vi "DumpToDashboard.vi"   [LabVIEW 2012]
uses:
  <vilib>/Rock Robotics/WPI/Joystick/WPI_JoystickGetSetRefNum.vi
types:
  T1 = typedef "WPI_JoystickDevRef.ctl" = cluster{"Device":T2}
  T2 = typedef "WPI_JoystickDeviceEnum.ctl" = enum16{"USB 1", "USB 2", "USB 3", "USB 4", "Kinect 1", "Kinect 2"}
  T3 = typedef "WPI_JoystickButtonState.ctl" = cluster{"Button 1":bool, "Button 2":bool, "Button 3":bool, "Button 4":bool, "Button 5":bool, "Button 6":bool, "Button 7":bool, "Button 8":bool, "Button 9":bool, "Button 10":bool, "Button 11":bool, "Button 12":bool}
  T4 = cluster{"axis 1 (x)":dbl, "axis 2 (y)":dbl, "axis 3 (throttle)":dbl, "axis 4":dbl, "axis 5":dbl, "axis 6":dbl}
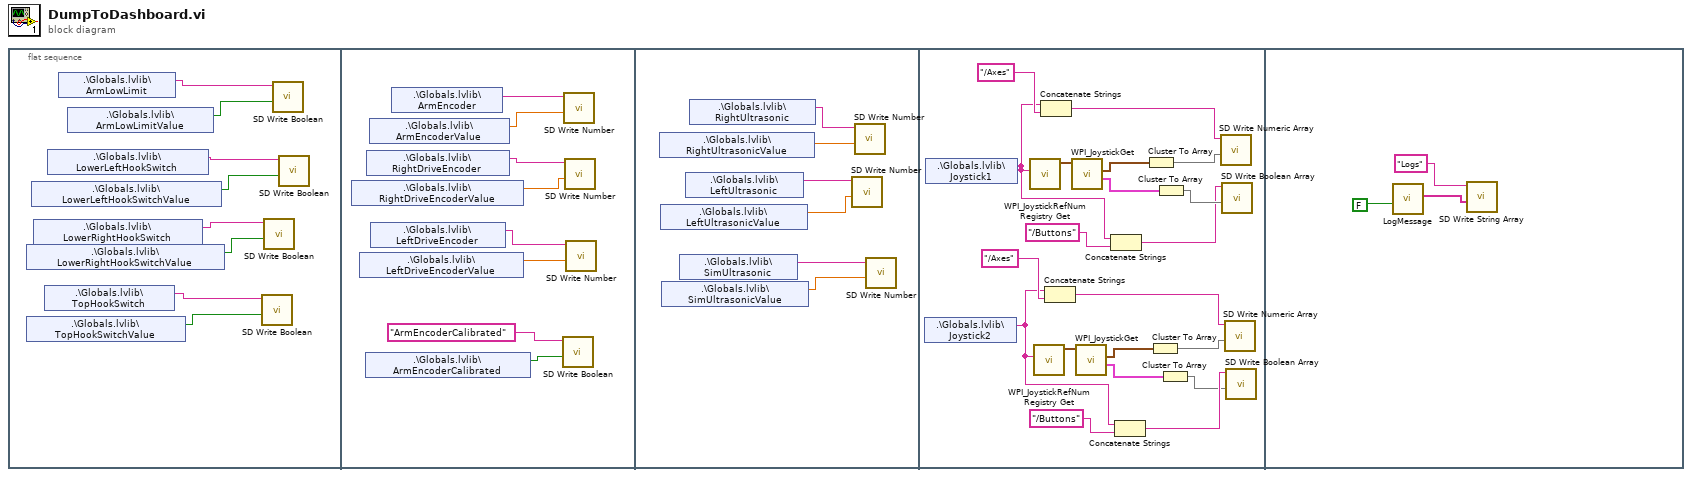
[diagram p0: block diagram]
diagram:
  n1 = flat-sequence {
    frame #0 {
      n2 = shared-variable ".\\Globals.lvlib\\LowerRightHookSwitchValue"() -> (w2:bool)  [unwired: 1 in, 1 out]
      n3 = shared-variable ".\\Globals.lvlib\\TopHookSwitchValue"() -> (w1:bool)  [unwired: 1 in, 1 out]
      n4 = shared-variable ".\\Globals.lvlib\\LowerLeftHookSwitchValue"() -> (w3:bool)  [unwired: 1 in, 1 out]
      n5 = shared-variable ".\\Globals.lvlib\\LowerRightHookSwitch"() -> (w6:string)  [unwired: 1 in, 1 out]
      n6 = shared-variable ".\\Globals.lvlib\\TopHookSwitch"() -> (w7:string)  [unwired: 1 in, 1 out]
      n7 = shared-variable ".\\Globals.lvlib\\LowerLeftHookSwitch"() -> (w5:string)  [unwired: 1 in, 1 out]
      n8 = shared-variable ".\\Globals.lvlib\\ArmLowLimit"() -> (w8:string)  [unwired: 1 in, 1 out]
      n9 = shared-variable ".\\Globals.lvlib\\ArmLowLimitValue"() -> (w4:bool)  [unwired: 1 in, 1 out]
      n10 = call <vilib>:"SD Write Boolean.vi"("Boolean"=w1, "Name"=w7) -> ()  [unwired: 8 in, 2 out]
      n11 = call <vilib>:"SD Write Boolean.vi"("Boolean"=w2, "Name"=w6) -> ()  [unwired: 8 in, 2 out]
      n12 = call <vilib>:"SD Write Boolean.vi"("Boolean"=w4, "Name"=w8) -> ()  [unwired: 8 in, 2 out]
      n13 = call <vilib>:"SD Write Boolean.vi"("Boolean"=w3, "Name"=w5) -> ()  [unwired: 8 in, 2 out]
    }
    frame #1 {
      n14 = shared-variable ".\\Globals.lvlib\\RightDriveEncoderValue"() -> (w13:dbl)  [unwired: 1 in, 1 out]
      n15 = shared-variable ".\\Globals.lvlib\\LeftDriveEncoderValue"() -> (w11:dbl)  [unwired: 1 in, 1 out]
      n16 = shared-variable ".\\Globals.lvlib\\ArmEncoderCalibrated"() -> (w10:bool)  [unwired: 1 in, 1 out]
      n17 = shared-variable ".\\Globals.lvlib\\RightDriveEncoder"() -> (w14:string)  [unwired: 1 in, 1 out]
      n18 = shared-variable ".\\Globals.lvlib\\ArmEncoderValue"() -> (w16:dbl)  [unwired: 1 in, 1 out]
      n19 = shared-variable ".\\Globals.lvlib\\LeftDriveEncoder"() -> (w12:string)  [unwired: 1 in, 1 out]
      n20 = shared-variable ".\\Globals.lvlib\\ArmEncoder"() -> (w15:string)  [unwired: 1 in, 1 out]
      n21 = call <vilib>:"SD Write Boolean.vi"("Boolean"=w10, "Name"="ArmEncoderCalibrated") -> ()  [unwired: 8 in, 2 out]
      n22 = call <vilib>:"SD Write Number.vi"("Numeric"=w16, "Name"=w15) -> ()  [unwired: 8 in, 2 out]
      n23 = call <vilib>:"SD Write Number.vi"("Numeric"=w13, "Name"=w14) -> ()  [unwired: 8 in, 2 out]
      n24 = call <vilib>:"SD Write Number.vi"("Numeric"=w11, "Name"=w12) -> ()  [unwired: 8 in, 2 out]
    }
    frame #2 {
      n25 = shared-variable ".\\Globals.lvlib\\RightUltrasonicValue"() -> (w21:dbl)  [unwired: 1 in, 1 out]
      n26 = shared-variable ".\\Globals.lvlib\\LeftUltrasonicValue"() -> (w19:dbl)  [unwired: 1 in, 1 out]
      n27 = shared-variable ".\\Globals.lvlib\\SimUltrasonicValue"() -> (w17:dbl)  [unwired: 1 in, 1 out]
      n28 = shared-variable ".\\Globals.lvlib\\SimUltrasonic"() -> (w18:string)  [unwired: 1 in, 1 out]
      n29 = shared-variable ".\\Globals.lvlib\\LeftUltrasonic"() -> (w20:string)  [unwired: 1 in, 1 out]
      n30 = shared-variable ".\\Globals.lvlib\\RightUltrasonic"() -> (w22:string)  [unwired: 1 in, 1 out]
      n31 = call <vilib>:"SD Write Number.vi"("Numeric"=w19, "Name"=w20) -> ()  [unwired: 8 in, 2 out]
      n32 = call <vilib>:"SD Write Number.vi"("Numeric"=w21, "Name"=w22) -> ()  [unwired: 8 in, 2 out]
      n33 = call <vilib>:"SD Write Number.vi"("Numeric"=w17, "Name"=w18) -> ()  [unwired: 8 in, 2 out]
    }
    frame #3 {
      n34 = shared-variable ".\\Globals.lvlib\\Joystick2"() -> (w23:string)  [unwired: 1 in, 1 out]
      n35 = shared-variable ".\\Globals.lvlib\\Joystick1"() -> (w33:string)  [unwired: 1 in, 1 out]
      n36 = call <vilib>:"WPI_JoystickRefNum Registry Get.vi"("refnum name"=w33) -> ("JoystickDevRef"=w42:T1)  [unwired: 1 in, 9 out]
      n37 = call <vilib>:"WPI_JoystickRefNum Registry Get.vi"("refnum name"=w23) -> ("JoystickDevRef"=w24:T1)  [unwired: 1 in, 9 out]
      n38 = Concatenate Strings(w33, "/Axes") -> (w37:string)
      n39 = Concatenate Strings(w23, "/Axes") -> (w29:string)
      n40 = call <vilib>:"WPI_JoystickGet.vi"("JoystickDevRef"=w42) -> ("Buttons"=w40:T3, "Axes"=w41:T4)  [unwired: 1 in, 4 out]
      n41 = call <vilib>:"WPI_JoystickGet.vi"("JoystickDevRef"=w24) -> ("Buttons"=w26:T3, "Axes"=w25:T4)  [unwired: 1 in, 4 out]
      n42 = Concatenate Strings(w33, "/Buttons") -> (w34:string)
      n43 = Concatenate Strings(w23, "/Buttons") -> (w32:string)
      n44 = Cluster To Array(cluster=w41) -> (array=w39:dbl[])
      n45 = Cluster To Array(cluster=w25) -> (array=w27:dbl[])
      n46 = Cluster To Array(cluster=w40) -> (array=w36:bool[])
      n47 = Cluster To Array(cluster=w26) -> (array=w30:bool[])
      n48 = call <vilib>:"SD Write Numeric Array.vi"("Numeric Array"=w39, "Name"=w37) -> ()  [unwired: 8 in, 2 out]
      n49 = call <vilib>:"SD Write Boolean Array.vi"("Boolean Array"=w36, "Name"=w34) -> ()  [unwired: 8 in, 2 out]
      n50 = call <vilib>:"SD Write Numeric Array.vi"("Numeric Array"=w27, "Name"=w29) -> ()  [unwired: 8 in, 2 out]
      n51 = call <vilib>:"SD Write Boolean Array.vi"("Boolean Array"=w30, "Name"=w32) -> ()  [unwired: 8 in, 2 out]
    }
    frame #4 {
      n52 = call "LogMessage.vi"("Log?"=FALSE) -> ("Logs"=w43:string[])  [unwired: 10 in]
      n53 = call <vilib>:"SD Write String Array.vi"("String Array"=w43, "Name"="Logs") -> ()  [unwired: 8 in, 2 out]
    }
  }
